vi "init.vi"(8 "error in (no error)":errorcluster, 11 "Protocol_TwoCreep in":refnum<class "Protocol_TwoCreep.lvclass">) -> (0 "error out":errorcluster, 3 "Protocol_TwoCreep out":refnum<class "Protocol_TwoCreep.lvclass">)   [LabVIEW 2011, in "Protocol_TwoCreep.lvclass"]
uses:
  Protocol_TwoCreep.lvclass
  protocol_Generic/Protocol_Generic.lvclass
  Protocol_TwoCreep.lvclass/Protocol_TwoCreep.ctl
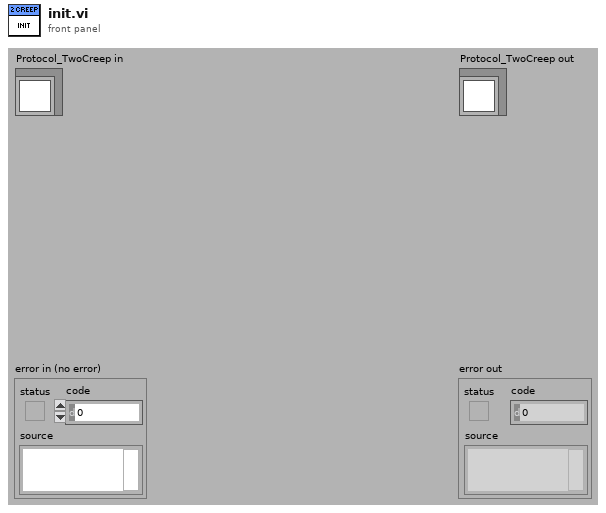
[diagram p1: front panel]
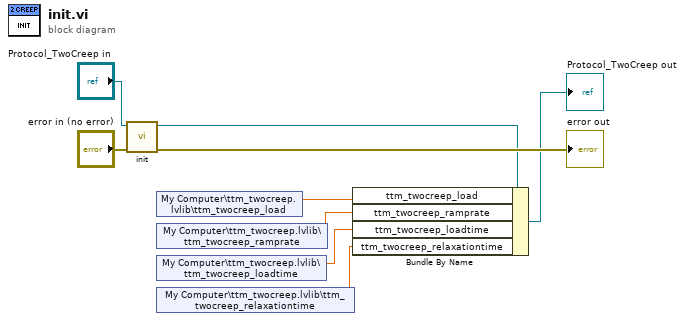
[diagram p0: block diagram]
diagram:
  n1 = call-parent "init.vi"("error in (no error)"="error in (no error)", "Protocol_Generic in"="Protocol_TwoCreep in") -> ("error out"=→"error out":errorcluster, "Protocol_Generic out"=w6:refnum<class "Protocol_TwoCreep.lvclass">)  [unwired: 8 in]
  n2 = shared-variable "My Computer\\ttm_twocreep.lvlib\\ttm_twocreep_load"() -> (w4:dbl)  [unwired: 1 in, 1 out]
  n3 = shared-variable "My Computer\\ttm_twocreep.lvlib\\ttm_twocreep_ramprate"() -> (w3:dbl)  [unwired: 1 in, 1 out]
  n4 = shared-variable "My Computer\\ttm_twocreep.lvlib\\ttm_twocreep_loadtime"() -> (w2:dbl)  [unwired: 1 in, 1 out]
  n5 = shared-variable "My Computer\\ttm_twocreep.lvlib\\ttm_twocreep_relaxationtime"() -> (w1:dbl)  [unwired: 1 in, 1 out]
  n6 = Bundle By Name(cluster=w6, "ttm_twocreep_load"=w4, "ttm_twocreep_ramprate"=w3, "ttm_twocreep_loadtime"=w2, "ttm_twocreep_relaxationtime"=w1) -> (→"Protocol_TwoCreep out":refnum<class "Protocol_TwoCreep.lvclass">)
